vi "Is_VI_Running.vi"(0 "Other_VI_Reference_In":refnum<vi>, 5 "This_VI_Reference_In":refnum<vi>, 11 "Error_In":errorcluster) -> (4 "Other_VI_Reference_Out":refnum<vi>, 6 "This_VI_Reference_Out":refnum<vi>, 8 "Stop":bool=TRUE, 15 "Error_Out":errorcluster)   [LabVIEW 2021]
doc: "Check if the VI running"
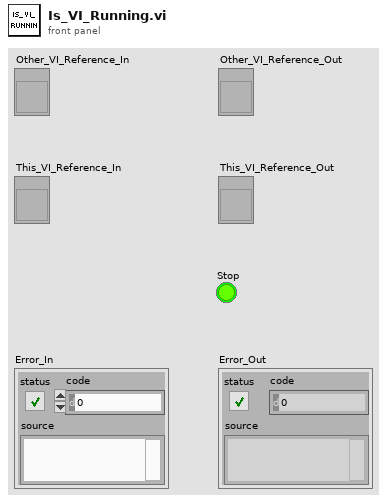
[diagram p1: front panel]
types:
  T1 = enum32{"Invalid", "Standard", "Closed", "Hidden", "Minimized", "Maximized"}
  T2 = enum32{"Bad", "Idle", "Run top level", "Running"}
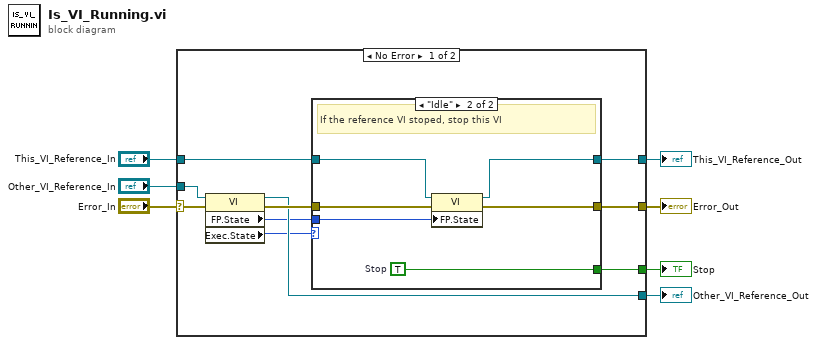
[diagram p0: block diagram]
diagram:
  n1 = case shown="No Error" "Error_In" {
    selector: "Error_In" -> [w16 w28]
    tunnel: "Other_VI_Reference_In" -> [w17 w27]
    tunnel: [w14 w28] -> w5
    tunnel: [w12 w27] -> w4
    tunnel: [w13 _] -> w3
    tunnel: "This_VI_Reference_In" -> [w11 w26]
    tunnel: [w10 w26] -> w1
    frame No Error {
      n2 = property class="VI"(reference=w17, error in=w16) -> (reference out=w12:refnum<vi>, error out=w15:errorcluster, "FP.State"=w8:T1, "Exec.State"=w9:T2)
      n3 = case shown="\"Idle\"" w9 {
        tunnel: w15 -> [w19 w24]
        tunnel: [w19 w23] -> w14
        tunnel: [_ w25] -> w13
        tunnel: w11 -> [w18 w22]
        tunnel: [w18 w21] -> w10
        tunnel: w8 -> [_ w20]
        frame "Running", Default {
        }
        frame "Idle" {
          w25 = TRUE  # Stop
          # "If the reference VI stoped, stop this VI"
          n4 = property class="VI"(reference=w22, error in=w24, "FP.State"=w20) -> (reference out=w21:refnum<vi>, error out=w23:errorcluster)
        }
      }
    }
    frame Error {
    }
  }
  "Error_Out" <- w5
  "Other_VI_Reference_Out" <- w4
  "Stop" <- w3
  "This_VI_Reference_Out" <- w1
